vi "Main - Interrupt Process.vi"(8 "error in (no error)":errorcluster, 10 "Queue Name":string) -> (0 "error out":errorcluster)   [LabVIEW 2011]
doc: "This is a basic Queue Driven Message Handler VI. Most advanced LabVIEW programmers who code extensively in LabVIEW utilitze some variation of this VI. This is a starting point. Some key features need to be added. In particular a robust error handling routine should be added.\n\nAAL 9/09"
uses:
  Shared/QDMH Poly VIs/QDMH POLY Enqueue String.vi
panel:
  in  "Interrupt Process":bool
  out "Message Display":string
  in  "Cancel":bool
  in  "OK":bool
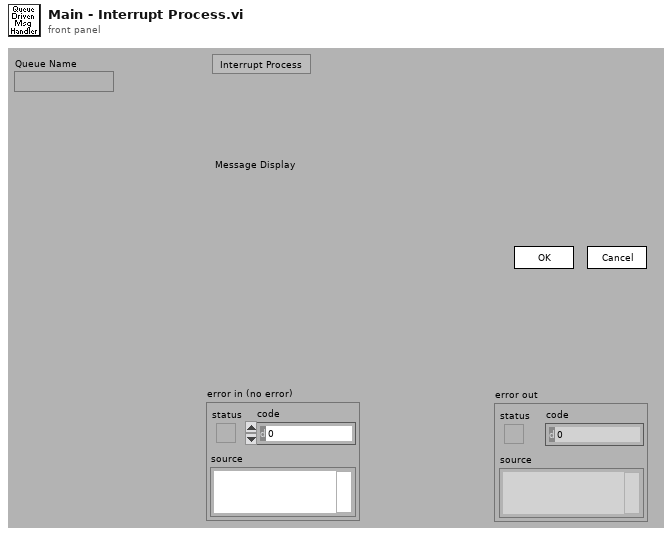
[diagram p1: front panel]
types:
  T1 = cluster{"Operator Name":string, "Current VI's Path":path, "Current VI's  Directory":path, "Queue Names":string[], "# VIs Launched":i32}
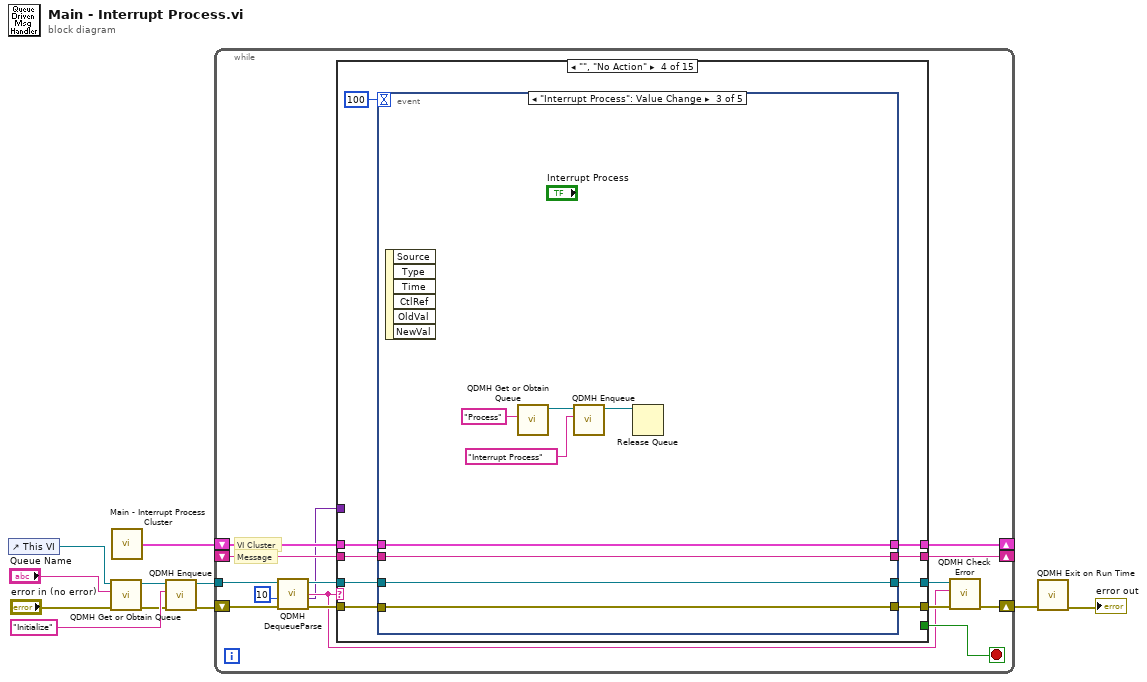
[diagram p0: block diagram]
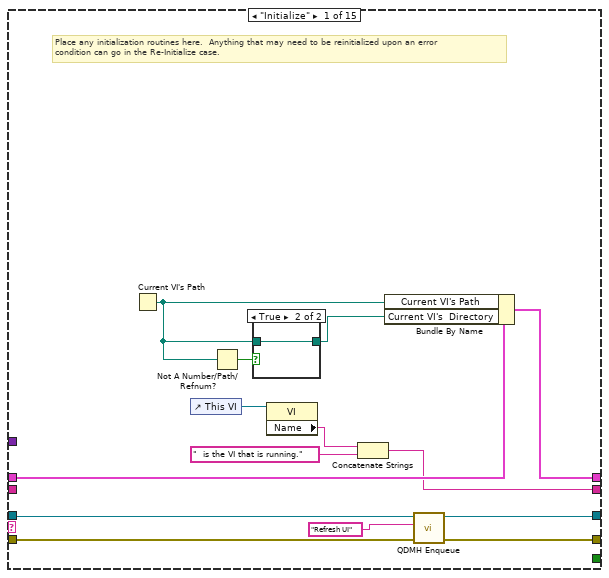
[diagram p2: hidden frame]
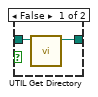
[diagram p3: hidden frame]
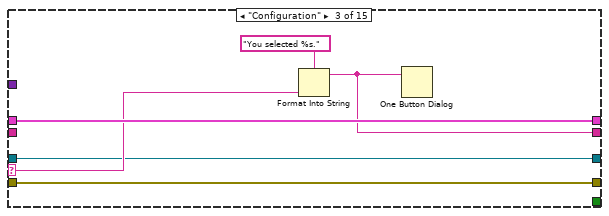
[diagram p5: hidden frame]
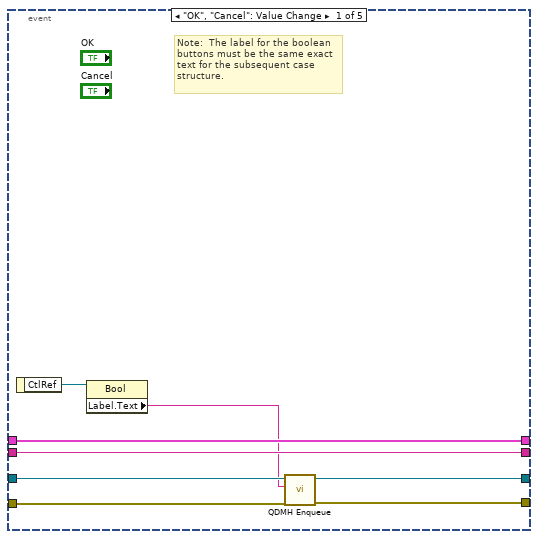
[diagram p6: hidden frame]
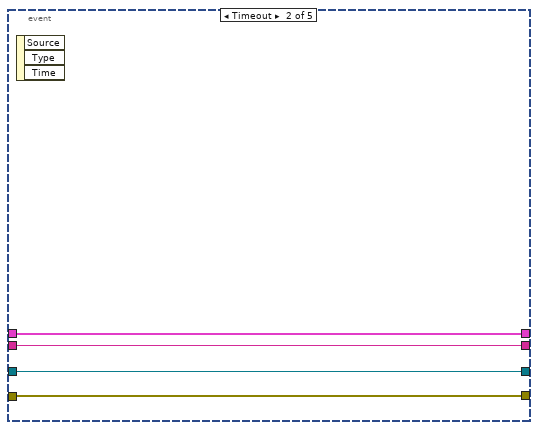
[diagram p7: hidden frame]
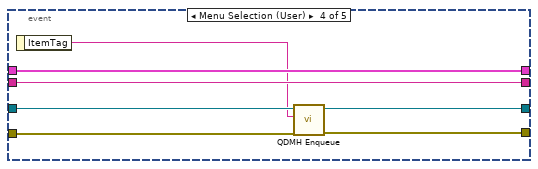
[diagram p8: hidden frame]
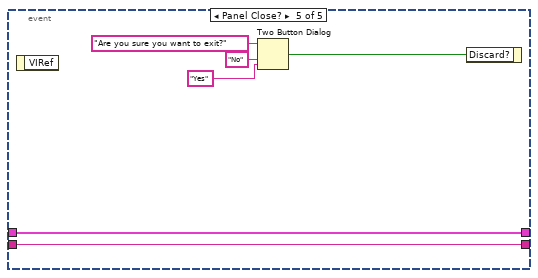
[diagram p9: hidden frame]
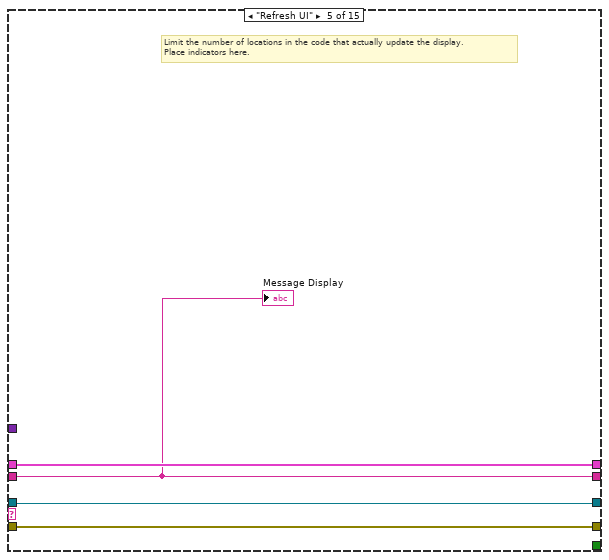
[diagram p10: hidden frame]
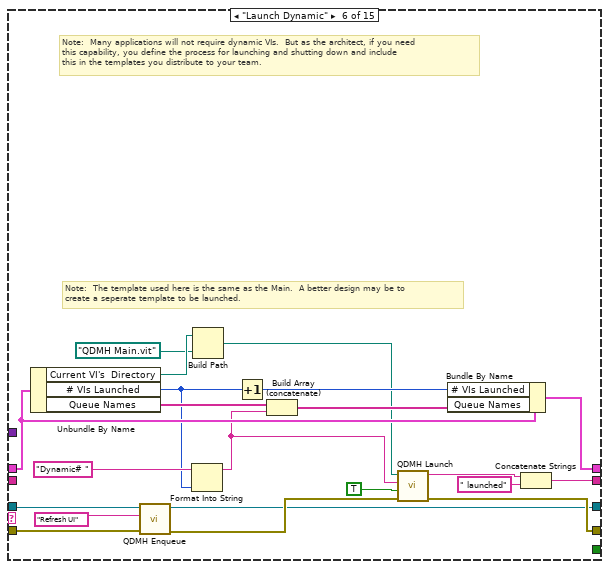
[diagram p11: hidden frame]
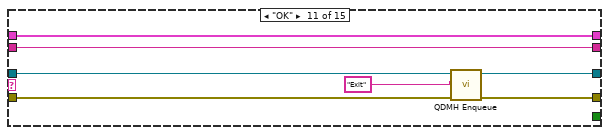
[diagram p16: hidden frame]
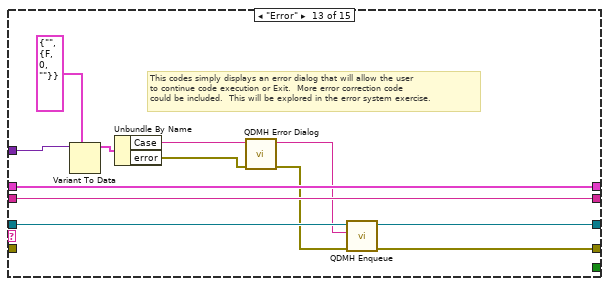
[diagram p18: hidden frame]
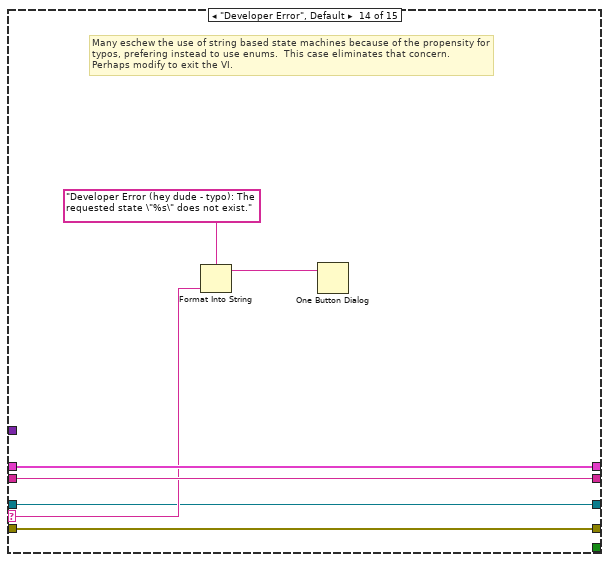
[diagram p19: hidden frame]
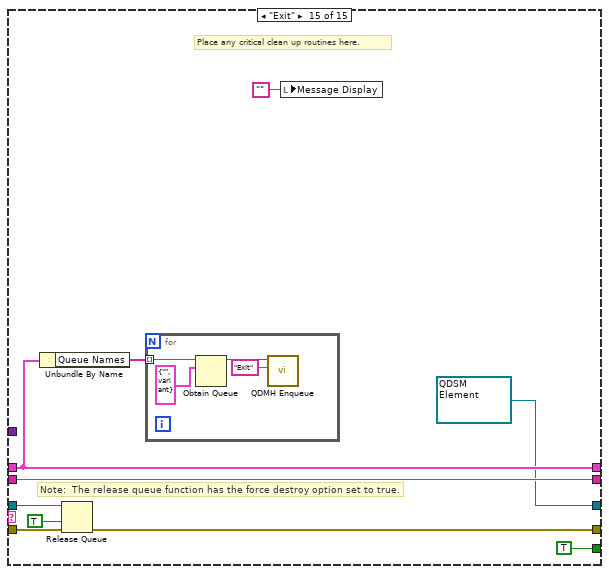
[diagram p20: hidden frame]
diagram:
  n1 = control-ref of="This VI"() -> (w3:refnum<vi>)
  n2 = call "QDMH Get or Obtain Queue.vi"("error in (no error)"="error in (no error)", "Queue Name"="Queue Name", "VI Refnum"=w3) -> ("error out"=w6:errorcluster, "queue out"=w7:refnum<queue>)  [unwired: 7 out]
  n3 = call "Main - Interrupt Process Cluster.vi"() -> ("Cluster"=w11:T1)
  n4 = call-poly "QDMH Enqueue.vi"("error in (no error)"=w6, "State"="Initialize" ("element"), "queue"=w7) -> ("error out"=w4:errorcluster, "queue out"=w5:refnum<queue>)  [unwired: 7 out]
  n5 = while {
    tunnel: w5 -> [w21]
    shift-left: w11 -> [w22]
    shift-right: [w23] -> _
    shift-left: _ -> [w24]
    shift-right: [w25] -> _
    shift-right: [w15] -> w2
    shift-left: w4 -> [w17]
    stop <- w26 stop-if-true
    # "VI Cluster"
    # "Message"
    n6 = call "QDMH DequeueParse.vi"("error in (no error)"=w17, "Timeout"=10 ("ms timeout (-1)"), "queue"=w21) -> ("error out"=w18:errorcluster, "Variant Data"=w12:variant, "State"=w13:string, "queue out"=w19:refnum<queue>)  [unwired: 5 out]
    n7 = case shown="\"\", \"No Action\"" w13 {
      selector: w13 -> [_ _ w50 _ _ _ _ _ _ _ _ _ _ w163 _]
      tunnel: w19 -> [w36 w44 w49 w62 w97 w116 w121 w125 w129 w133 w143 w145 w157 w160 w173]
      tunnel: [_ _ _ _ _ _ _ _ _ _ _ _ _ _ TRUE] -> w26
      tunnel: [w34 w47 w51 w55 w98 w117 w124 w128 w132 w136 w142 w147 w159 w166 w175] -> w25
      tunnel: w24 -> [_ w47 _ w56 w98 _ w124 w128 w132 w136 w142 w147 w159 w166 w175]
      tunnel: [w39 w46 w53 w57 w99 w113 w123 w127 w131 w135 w141 w146 w158 w165 w170] -> w23
      tunnel: w22 -> [w40 w46 w53 w58 w99 w114 w123 w127 w131 w135 w141 w146 w158 w165 w170]
      tunnel: w18 -> [w38 w45 w48 w61 w96 w107 w122 w126 w130 w134 w140 w144 _ w162 w172]
      tunnel: [w37 w45 w48 w60 w96 w106 w122 w126 w130 w134 w139 w144 w156 w162 w167] -> w16
      tunnel: [w29 w44 w49 w54 w97 w103 w121 w125 w129 w133 w137 w145 w155 w160 refnum<queue> refnum ("queue out")] -> w14
      tunnel: w12 -> [_ _ _ _ _ _ _ _ _ _ _ _ w153 _ _]
      frame "Initialize" {
        # "Place any initialization routines here.  Anything that may need to be reinitialized upon an error\ncondition can go in the Re-Initialize case."
        n8 = Current VI's Path() -> (path=w27:path)
        n9 = control-ref of="This VI"() -> (w33:refnum<vi>)
        n10 = Not A Number/Path/Refnum?(number/path/refnum=w27) -> (NaN/Path/Refnum?=w28:bool)
        n11 = case shown="True" w28 {
          tunnel: w27 -> [w42 w43]
          tunnel: [w41 w43] -> w31
          frame False {
            n12 = call "UTIL Get Directory.vi"("Path In"=w42) -> ("Directory Out"=w41:path)  [unwired: 1 in, 9 out]
          }
          frame True {
          }
        }
        n13 = property class="VI"(reference=w33) -> ("Name"=w32:string)  [unwired: 1 in, 2 out]
        n14 = Concatenate Strings(w32, "  is the VI that is running." ("string")) -> (w34:string)
        n15 = Bundle By Name(cluster=w40, "Current VI's Path"=w27, "Current VI's  Directory"=w31) -> (w39:T1)
        n16 = call-poly "QDMH Enqueue.vi"("error in (no error)"=w38, "State"="Refresh UI" ("New State"), "queue"=w36) -> ("error out"=w37:errorcluster, "queue out"=w29:refnum<queue>)  [unwired: 7 out]
      }
      frame "Re-Initialize" {
        # "This case includes initialization functionality that may need to run again during the course of the VI"
      }
      frame "Configuration" {
        n17 = Format Into String(format string="You selected %s." ("Format String"), w50) -> (resulting string=w51:string)  [unwired: 2 in, 1 out]
        n18 = One Button Dialog(message=w51) -> ()  [unwired: 2 out]
      }
      frame "", "No Action" {
        n19 = event shown="[2] \"Interrupt Process\": Value Change" {
          selector: _ -> [_ _ _ _ _]
          dyn-events: _ -> [_ _ _ _ _]
          timeout: 100 -> [_ _ _ _ _]
          tunnel: w62 -> [w69 w71 w79 w89 _]
          tunnel: [w68 w74 w82 w87 _] -> w60
          tunnel: w61 -> [w67 w74 w82 w88 _]
          tunnel: w58 -> [w66 w73 w81 w86 w95]
          tunnel: [w66 w73 w81 w86 w95] -> w57
          tunnel: w56 -> [w65 w72 w80 w85 w94]
          tunnel: [w65 w72 w80 w85 w94] -> w55
          tunnel: [w63 w71 w79 w83 _] -> w54
          event "OK", "Cancel": Value Change {
            # "Note:  The label for the boolean buttons must be the same exact text for the subsequent case structure."
            n20 = event-data() -> ("CtlRef"=w70:refnum<vi>)  [unwired: 1 out]
            n21 = property class="Bool"(reference=w70) -> ("Label.Text"=w64:string)  [unwired: 1 in, 2 out]
            n22 = call-poly "QDMH Enqueue.vi"("error in (no error)"=w67, "State"=w64, "queue"=w69) -> ("error out"=w68:errorcluster, "queue out"=w63:refnum<queue>)  [unwired: 7 out]
          }
          event Timeout {
            n23 = event-data() -> ()  [unwired: 4 out]
          }
          event "Interrupt Process": Value Change {
            n24 = event-data() -> ()  [unwired: 7 out]
            n25 = call "QDMH Get or Obtain Queue.vi"("Queue Name"="Process") -> ("queue out"=w78:refnum<queue>)  [unwired: 2 in, 8 out]
            n26 = call-poly "QDMH Enqueue.vi"("State"="Interrupt Process" ("name (unnamed)"), "queue"=w78) -> ("queue out"=w75:refnum<queue>)  [unwired: 1 in, 8 out]
            n27 = Release Queue(queue=w75) -> ()  [unwired: 2 in, 3 out]
          }
          event Menu Selection (User) {
            n28 = event-data() -> ("ItemTag"=w84:string)  [unwired: 1 out]
            n29 = call-poly "QDMH Enqueue.vi"("error in (no error)"=w88, "State"=w84, "queue"=w89) -> ("error out"=w87:errorcluster, "queue out"=w83:refnum<queue>)  [unwired: 7 out]
          }
          event Panel Close? {
            n30 = event-data() -> ()  [unwired: 2 out]
            n31 = Two Button Dialog(message="Are you sure you want to exit?", 1:"Yes" ("F button name (\"Cancel\")"), 2:"No" ("T button name (\"OK\")")) -> (T button?=w90:bool)
            n32 = event-data("Discard?"=w90) -> ()  [unwired: 1 in, 1 out]
          }
        }
      }
      frame "Refresh UI" {
        # "Limit the number of locations in the code that actually update the display.\nPlace indicators here."
        "Message Display" <- w98
      }
      frame "Launch Dynamic" {
        # "Note:  The template used here is the same as the Main.  A better design may be to\ncreate a seperate template to be launched."
        # "Note:  Many applications will not require dynamic VIs.  But as the architect, if you need\nthis capability, you define the process for launching and shutting down and include\nthis in the templates you distribute to your team."
        n33 = Unbundle By Name(w114) -> ("Current VI's  Directory"=w102:path, "# VIs Launched"=w110:i32, "Queue Names"=w112:string[])
        n34 = call-poly "QDMH Enqueue.vi"("error in (no error)"=w107, "State"="Refresh UI" ("New State"), "queue"=w116) -> ("error out"=w105:errorcluster, "queue out"=w103:refnum<queue>)  [unwired: 7 out]
        n35 = Format Into String(initial string="Dynamic# ", w110) -> (resulting string=w108:string)  [unwired: 2 in, 1 out]
        n36 = Build Path(base path=w102, name or relative path=path "QDMH Main.vit" ("vi path")) -> (appended path=w100:path)
        n37 = Increment(x=w110) -> (x+1=w109:i32)
        n38 = Build Array (concatenate)(w112, w108) -> (w111:string[])
        n39 = call "QDMH Launch.vi"("error in (no error)"=w105, "Front Panel Window (Open)"=TRUE ("Front Panel Window:Open"), "Queue Name"=w108, "VI Path"=w100) -> ("error out"=w106:errorcluster, "Launched VI Name"=w119:string)  [unwired: 6 out]
        n40 = Bundle By Name(cluster=w114, "# VIs Launched"=w109, "Queue Names"=w111) -> (w113:T1)
        n41 = Concatenate Strings(w119, " launched" ("string")) -> (w117:string)
      }
      frame "Shutdown Dynamic" {
      }
      frame "Send Message to Dynamic" {
      }
      frame "Receive Message From Dynamic" {
      }
      frame "<duplicate me for new states >" {
        # "Duplicate this state for any additional states that you add."
      }
      frame "OK" {
        n42 = call-poly "QDMH Enqueue.vi"("error in (no error)"=w140, "State"="Exit" ("New State"), "queue"=w143) -> ("error out"=w139:errorcluster, "queue out"=w137:refnum<queue>)  [unwired: 7 out]
      }
      frame "Cancel" {
      }
      frame "Error" {
        # "This codes simply displays an error dialog that will allow the user\nto continue code execution or Exit.  More error correction code\ncould be included.  This will be explored in the error system exercise."
        n43 = Variant To Data(type=cluster{"Case":string, "error":errorcluster} {"Case"="", "error"={"status"=FALSE, "code"=0, "source"=""}} ("QDSM Element"), Variant=w153) -> (data=w152:cluster{"Case":string, "error":errorcluster})  [unwired: 1 in, 1 out]
        n44 = Unbundle By Name(w152) -> ("Case"=w151:string, "error"=w150:errorcluster)
        n45 = call "QDMH Error Dialog.vi"("error"=w150, "Case Error Occured"=w151) -> ("error out (no error)"=w148:errorcluster, "Case to Execute"=w149:string)  [unwired: 8 out]
        n46 = call-poly "QDMH Enqueue.vi"("error in (no error)"=w148, "State"=w149, "queue"=w157) -> ("error out"=w156:errorcluster, "queue out"=w155:refnum<queue>)  [unwired: 7 out]
      }
      frame "Developer Error", Default {
        # "Many eschew the use of string based state machines because of the propensity for\ntypos, prefering instead to use enums.  This case eliminates that concern.\nPerhaps modify to exit the VI."
        n47 = Format Into String(format string="Developer Error (hey dude - typo): The requested state \"%s\" does not exist." ("message"), w163) -> (resulting string=w161:string)  [unwired: 2 in, 1 out]
        n48 = One Button Dialog(message=w161) -> ()  [unwired: 2 out]
      }
      frame "Exit" {
        # "Note:  The release queue function has the force destroy option set to true."
        # "Place any critical clean up routines here."
        n49 = Unbundle By Name(w170) -> ("Queue Names"=w168:string[])
        n50 = Release Queue(queue=w173, force destroy? (F)=TRUE, error in (no error)=w172) -> (error out=w167:errorcluster)  [unwired: 2 out]
        n51 = for {
          tunnel: w168 -> [w180] mode=indexing
          n52 = Obtain Queue(name (unnamed)=w180, element data type=cluster{"State":string, "Variant Data":variant} {"State"="", "Variant Data"=variant} ("QDSM Element")) -> (queue out=w179:refnum<queue>)  [unwired: 3 in, 2 out]
          n53 = call-poly "QDMH Enqueue.vi"("State"="Exit" ("element"), "queue"=w179) -> ()  [unwired: 1 in, 9 out]
        }
        n54 = local write "Message Display"("") -> ()
      }
    }
    n55 = call "QDMH Check Error.vi"("error in (no error)"=w16, "Case"=w13, "queue"=w14) -> ("error out"=w15:errorcluster)  [unwired: 1 in, 7 out]
  }
  n56 = call "QDMH Exit on Run Time.vi"("error in (no error)"=w2) -> ("error out"=→"error out":errorcluster)  [unwired: 10 in]
